vi "Create Group.vi"(4 "Channel Resources (Unset)":string[](array[string]), 5 "Raw Values (F)":bool, 6 "Channel Names":string[](array[string]), 7 "Group Type":refnum<class "GroupAbstract.lvclass">, 8 "error in (no error)":errorcluster, 9 "Publish Config (Local Only)":T1, 10 "Group Name":string, 11 "Module in":refnum<class "Module.lvclass">) -> (0 "error out":errorcluster, 2 "Group":refnum<class "GroupAbstract.lvclass">, 3 "Module out":refnum<class "Module.lvclass">)   [LabVIEW 2020, in "Volatus.lvlib" / "Module.lvclass"]
uses:
  Module.lvclass
  lv-vecto/Vecto/GroupAbstract/GroupAbstract.lvclass
  lv-vecto/Vecto/Publish Config.ctl
  lv-vecto/Vecto/Group Info.ctl
  Module.lvclass/Module.ctl
  lv-vecto/Vecto/Vecto.lvlib
  VolatusAPI/VolatusAPI.lvclass
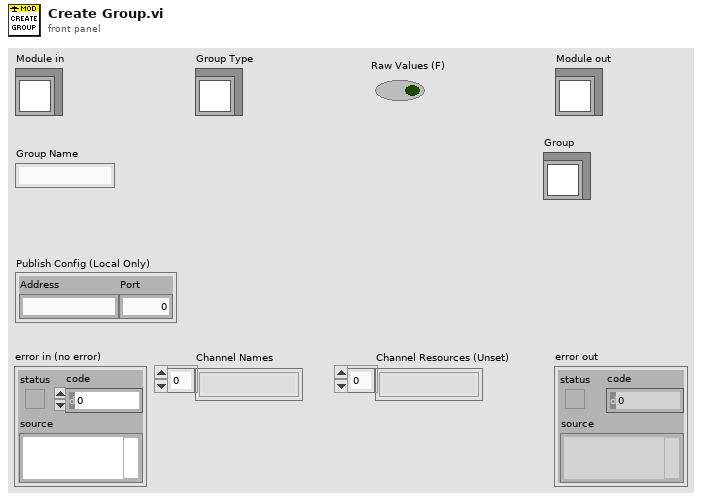
[diagram p1: front panel]
types:
  T1 = typedef "Vecto.lvlib/Publish Config.ctl" = cluster{"Address":string, "Port":u16}
  T2 = typedef "Vecto.lvlib/Group Info.ctl" = cluster{"System":string, "Cluster":string, "Node":string, "Task":string, "Name":string}
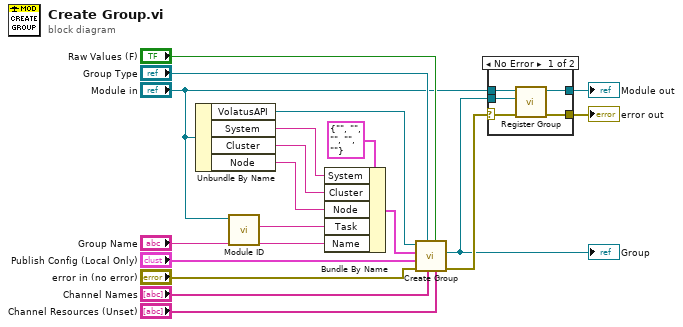
[diagram p0: block diagram]
diagram:
  n1 = Unbundle By Name("Module in") -> ("VolatusAPI"=w10:refnum<class "VolatusAPI.lvclass">, "System"=w16:string, "Cluster"=w15:string, "Node"=w14:string)
  n2 = call-dynamic "Module ID.vi"("Module in"="Module in") -> ("Module ID"=w2:string)  [unwired: 10 in]
  n3 = Bundle By Name(cluster=T2 {"System"="", "Cluster"="", "Node"="", "Task"="", "Name"=""} ("Group Info"), "System"=w16, "Cluster"=w15, "Node"=w14, "Task"=w2, "Name"="Group Name") -> (w11:T2)
  n4 = call "Create Group.vi"("Channel Resources (Unset)"="Channel Resources (Unset)", "Raw Values (F)"="Raw Values (F)", "Channel Names"="Channel Names", "Group Type"="Group Type", "error in (no error)"="error in (no error)", "Publish Config (None)"="Publish Config (Local Only)", "Group Info"=w11, "VolatusAPI in"=w10) -> ("error out"=w19:errorcluster, "Group"=w4:refnum<class "GroupAbstract.lvclass">)  [unwired: 1 in, 1 out]
  "Group" <- w4
  n5 = case shown="No Error" w19 {
    selector: w19 -> [w20 w26]
    tunnel: "Module in" -> [w24 w25]
    tunnel: [w23 w25] -> w18
    tunnel: [w22 w26] -> w3
    tunnel: w4 -> [w21 _]
    frame No Error {
      n6 = call "Register Group.vi"("error in (no error)"=w20, "Group"=w21, "Module in"=w24) -> ("error out"=w22:errorcluster, "Module out"=w23:refnum<class "Module.lvclass">)  [unwired: 7 in]
    }
    frame Error {
    }
  }
  "error out" <- w3
  "Module out" <- w18
